vi "monthwise_bd_summery.vi"(8 "O/P 3":string[](array[string]), 9 "error in (no error)":errorcluster, 11 "Table":string[][](array[string])) -> (1 "error out":errorcluster, 2 "O/P 2":string[](array[string]), 3 "O/P":string[](array[string]))   [LabVIEW 2017]
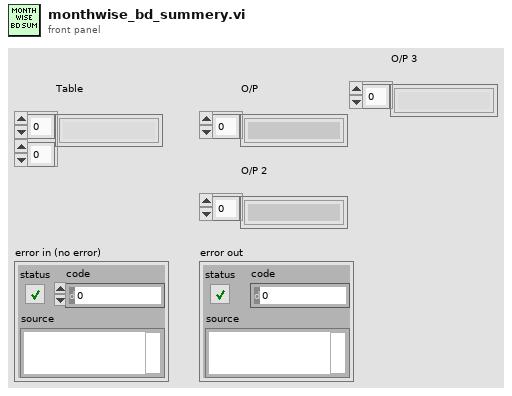
[diagram p1: front panel]
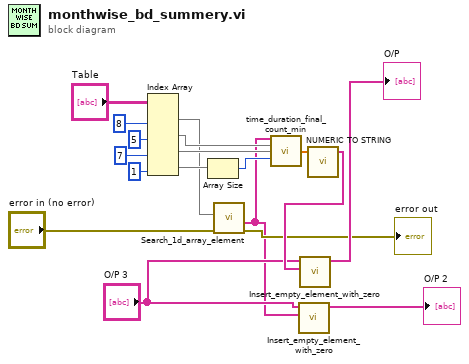
[diagram p0: block diagram]
diagram:
  n1 = Index Array(array="Table", index (col) #1=8 ("disabled index (col)"), index (col) #2=5 ("disabled index (col)"), index (col) #3=7 ("disabled index (col)"), index (col) #4=1 ("disabled index (col)")) -> (element #1=w4:string[], element #2=w8:string[], element #3=w9:string[], element #4=w13:string[])  [unwired: 4 in]
  n2 = Array Size(array=w13) -> (size(s)=w11:i32)
  n3 = call "Search_1d_array_element.vi"("error in (no error)"="error in (no error)", "BD Date"=w4) -> ("error out"=→"error out":errorcluster, "Count out"=w1:string[])  [unwired: 5 in, 1 out]
  n4 = call "time_duration_final_count_min.vi"("BD Count"=w1, "Intime"=w8, "OutTime"=w9, "bd array size"=w11) -> ("appended array"=w16:dbl[])  [unwired: 8 in, 3 out]
  n5 = call "Insert_empty_element_with_zero.vi"("searched date"=w1, "fixed date"="O/P 3") -> ("O/P"=→"O/P 2":string[])  [unwired: 9 in]
  n6 = call "NUMERIC TO STRING.vi"("appended array"=w16) -> ("Array"=w15:string[])  [unwired: 4 in]
  n7 = call "Insert_empty_element_with_zero.vi"("searched date"=w15, "fixed date"="O/P 3") -> ("O/P"=→"O/P":string[])  [unwired: 9 in]
